vi "Test Schnittpunkte.vi"() -> ()   [LabVIEW 2019]
uses:
  Gerade/Gerade.lvclass
panel:
  out "Sensor auf Linie":bool=TRUE
  out "Schnittpunkt":dbl[](array[numeric])=[10.0, 0.375]
  out "XY Graph":cluster{"x":dbl[], "y":dbl[]}[](graph)=[{"x"=[10.0, 10.0], "y"=[-10.0, 10.0]}, {"x"=[7.0, 15.0], "y"=[0.0, 1.0]}, {"x"=[10.0], "y"=[0.375]}]
  in  "Sensorkoord [P1 P2]":dbl[][](array[numeric])=[[7.0, 15.0], [0.0, 1.0]]
  in  "horizontal":bool
  in  "Endpunkt":dbl[](array[numeric])=[10.0, 10.0]
  in  "Startpunkt":dbl[](array[numeric])=[10.0, -10.0]
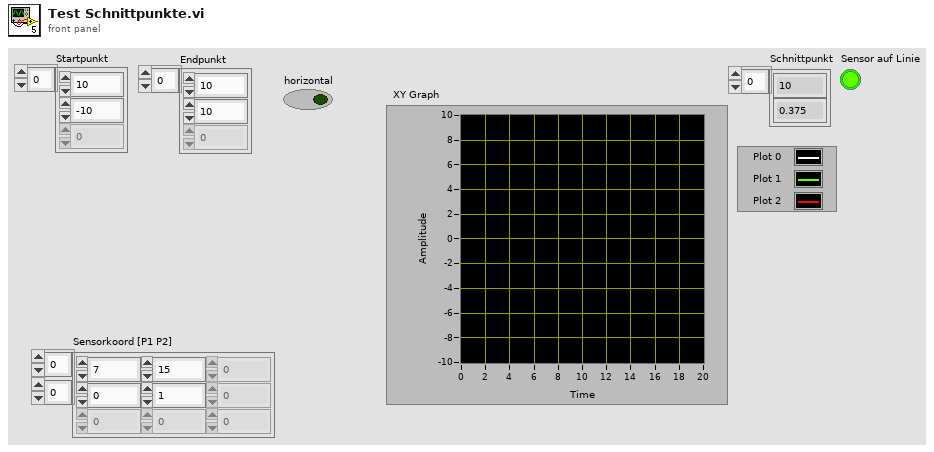
[diagram p1: front panel]
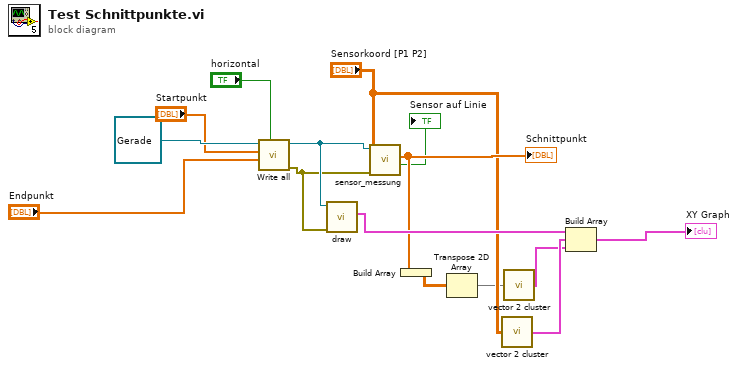
[diagram p0: block diagram]
diagram:
  n1 = call-dynamic "Write all.vi"("horizontal"="horizontal", "Endpunkt"="Endpunkt", "Startpunkt"="Startpunkt", "Gerade in"=refnum<class "Gerade.lvclass"> refnum ("Gerade.lvclass")) -> ("error out"=w10:errorcluster, "Gerade out"=w11:refnum<class "Gerade.lvclass">)  [unwired: 6 in]
  n2 = call-dynamic "draw.vi"("error in (no error)"=w10, "Gerade in"=w11) -> ("Line"=w9:cluster{"x":dbl[], "y":dbl[]})  [unwired: 7 in, 2 out]
  n3 = call-dynamic "sensor_messung.vi"("error in (no error)"=w10, "Sensorkoord [P1 P2]"="Sensorkoord [P1 P2]", "Gerade in"=w11) -> ("Sensor auf Linie"=→"Sensor auf Linie":bool, "Schnittpunkt"=w7:dbl[])  [unwired: 5 in, 2 out]
  "Schnittpunkt" <- w7
  n4 = Build Array(w7) -> (w6:dbl[][])
  n5 = Transpose 2D Array(2D array=w6) -> (transposed array=w1:dbl[][])
  n6 = call "vector 2 cluster.vi"("coordinates"="Sensorkoord [P1 P2]") -> (0:w3:cluster{"x":dbl[], "y":dbl[]})
  n7 = call "vector 2 cluster.vi"("coordinates"=w1) -> (0:w2:cluster{"x":dbl[], "y":dbl[]})
  n8 = Build Array(w9, w3, w2) -> (→"XY Graph":cluster{"x":dbl[], "y":dbl[]}[])
